vi "SubVI_NewPath.vi"(10 "Channel Selection":bool[](array[boolean]), 11 "source file path":path) -> (3 "New file path":path)   [LabVIEW 2011]
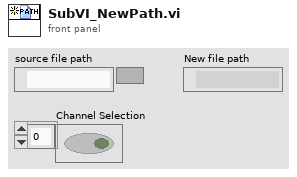
[diagram p1: front panel]
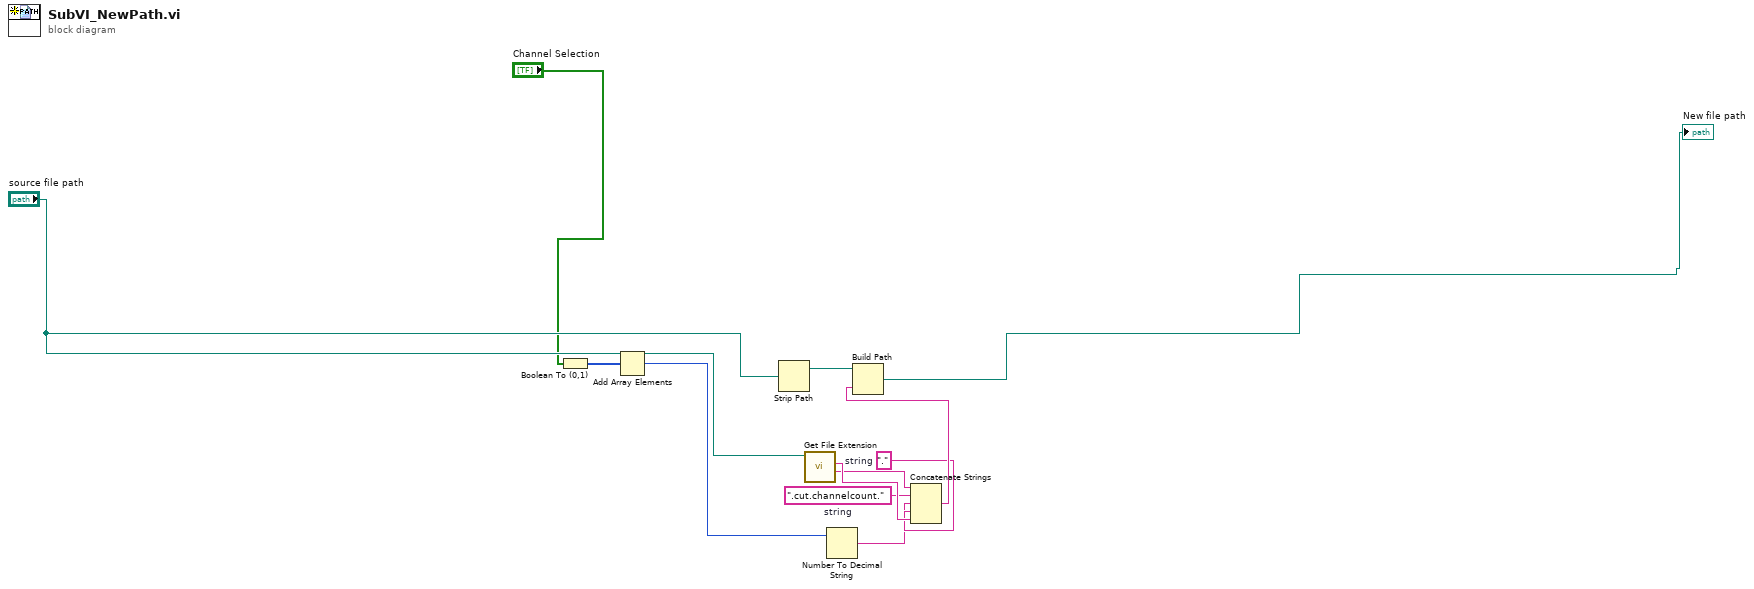
[diagram p0: block diagram]
diagram:
  w8 = "."  # string
  w5 = ".cut.channelcount."  # string
  n1 = Boolean To (0,1)(Boolean="Channel Selection") -> (0, 1=w2:i16[])
  n2 = Add Array Elements(numeric array=w2) -> (sum=w6:i16)
  n3 = Strip Path(path="source file path") -> (stripped path=w3:path)  [unwired: 1 out]
  n4 = call <vilib>:"Get File Extension.vi"("file"="source file path") -> ("filename without extension"=w4:string, "lowercase file extension"=w9:string)  [unwired: 7 in, 2 out]
  n5 = Number To Decimal String(number=w6) -> (decimal integer string=w7:string)  [unwired: 1 in]
  n6 = Concatenate Strings(w4, w5, w7, w8, w9) -> (w10:string)
  n7 = Build Path(base path=w3, name or relative path=w10) -> (appended path=→"New file path":path)
